vi "ImagerForFlowbit5.vi"() -> ()   [LabVIEW 2011]
uses:
  <vilib>/vision/Image Controls.llb/IMAQ Image.ctl
  <vilib>/Platform/TimedLoop/XDataNode/timing_clust.ctl
  <vilib>/Platform/TimedLoop/XDataNode/nitl_modes.ctl
  <vilib>/Platform/TimedLoop/XDataNode/wakeup.ctl
  <vilib>/Utility/config.llb/Read Key (I32).vi
  <vilib>/Analysis/1siggen.llb/Riffle Array (I32).vi
  <vilib>/Platform/TimedLoop/XDataNode/XDataNode.xnode
  <vilib>/Analysis/NI_AALBase.lvlib
  <vilib>/vision/NI_Vision_Development_Module.lvlib
  <vilib>/Platform/TimedLoop/XDataNode/XDNodeRunTimeDep.lvlib
  <vilib>/Utility/config.llb/NI_LVConfig.lvlib
panel:
  out "onLineMapOutput":T1[](array[typedef])
  out "Bounds.Right":i16
  out "停止循环":bool
  in  "Stimuli":i64=5
  in  "选项卡控件":enum32{"前面板", "参数设置", "OnLineMap"}(tab)
  out "log":string
  out "Stim_ID":i32(listbox)=1
  in  "开始/暂停":bool=TRUE
  in  "停止":bool
  out "重排的 Stim ID":i32[](array[numeric]) caption="重排的{X}"
  out "block":i32
  out "队列中元素数量":i32
  out "Image 2":T1(plugin-control)
  in  "热图":bool
  out "循环持续时间":i64
  out "Recording":bool
  out "grabLoop":i32
  out "writeing data":bool
  out "address":i16=888 caption="地址" format="%.0x"
  in  "SaveParameter":bool
  in  "Pra_binType":enum16{"Extract", "Resample"}(ring)
  in  "Pra_FramesPerStim":i64=16
  in  "Pra_Blk目录":path=path "D:/Expt/test"
  in  "Pra_文件名":string="G4_E02"
  in  "Pra_TimeForPrepare(ms)":u32=1000
  in  "Pra_stim ID":u8[](array[numeric])=[0, 2, 4, 6, 8]
  in  "Pra_blk总数":i32=500
  in  "Pra_stim protocol":T2(array[ring])=[enum."prep stim", enum."wait respirator", enum."show stim", enum."recording data", enum."Blank stim", enum."writing data", enum."ISI"]
  in  "Pra_blank stim":u8
  in  "Pra_wait（ms）":u32=10
  in  "Pra_ISI（ms）":u32=8000
  in  "Pra_FrameBin":i32=25
  in  "Pra_datatype":u16(ring)=13 items=["U8"=11, "I16"=12, "U32"=13, "SGL"=14]
  in  "FrameWidth":i64=704
  in  "FrameHeight":i64=576
  in  "LoadParameter":bool
  in  "Pra_bin":enum16{"1*1", "2*2"}(ring)
  in  "Pra_DR/R parameter":T3={"frame_zero_0"=0, "frame_zero_1"=1, "frame_0"=3, "frame_1"=15}
  in  "Pra_OnlineMap":cluster{"数组 1":i32[], "数组 2":i32[]}[](array[cluster])=[{"数组 1"=[2], "数组 2"=[6]}, {"数组 1"=[4], "数组 2"=[8]}, {"数组 1"=[2, 6], "数组 2"=[4, 8]}, {"数组 1"=[2, 4, 6, 8], "数组 2"=[0]}, {"数组 1"=[2, 4], "数组 2"=[6, 8]}]
  in  "Pra_clip ratio":dbl=2.0 min=0.0001 step=0.1
  # "-"
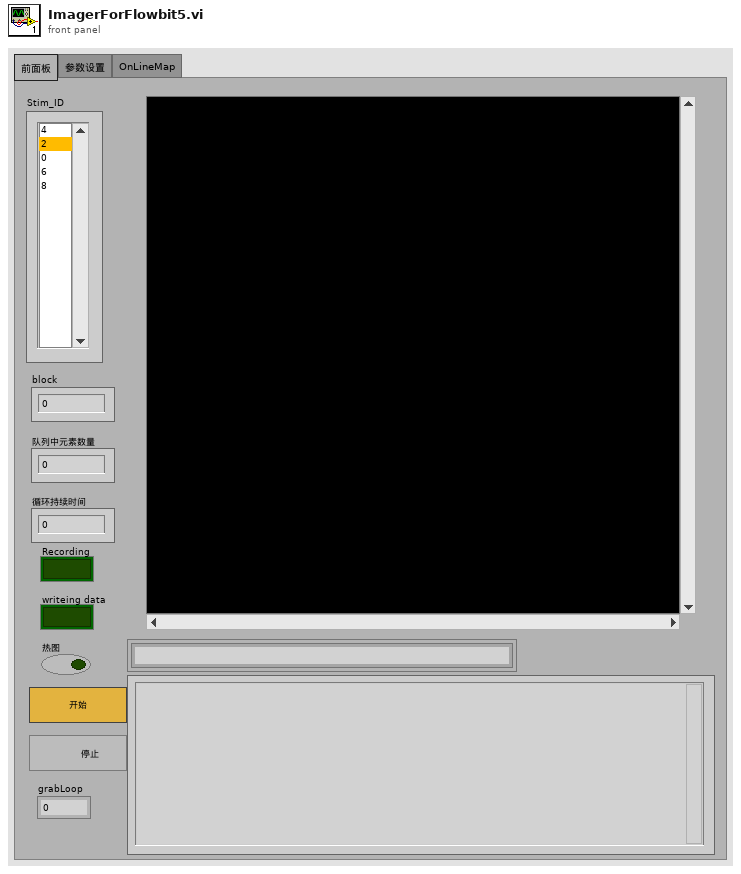
[diagram p1: front panel]
types:
  T1 = typedef "IMAQ Image.ctl" = refnum<image>
  T2 = enum16{"wait", "prep stim", "show stim", "wait respirator", "recording data", "Blank stim", "wait heart", "ISI", "DR/R", "wait calibrate", "openLightShutter", "closeLightShutter", "writing data"}[]
  T3 = cluster{"frame_zero_0":i32, "frame_zero_1":i32, "frame_0":i32, "frame_1":i32}
  T4 = typedef "Image Type" = u32
  T5 = enum16{"Disable External Trigger", "Enable External Trigger"}
  T6 = enum32{"Auto Detect", "RoadRunner", "Raven", "R64"}
  T7 = typedef "LVAllMonitorsDisplayTypeDef.ctl" = cluster{"Bounds":cluster{"Left":i16, "Top":i16, "Right":i16, "Bottom":i16}, "Depth":i16}[]
  T8 = cluster{"Bounds":cluster{"Left":i16, "Top":i16, "Right":i16, "Bottom":i16}, "Depth":i16}
  T9 = typedef "NI_LVConfig.lvlib/Config Data RefNum.ctl" = refnum<k1>
  T10 = enum16{"big-endian, network order", "native, host order", "little-endian"}
  T11 = enum8{"Enabled", "Disabled", "Disabled and Grayed Out"}
  T12 = enum16{"open", "replace", "create", "open or create", "replace or create", "replace or create with confirmation"}
  T13 = cluster{"Browser Size":cluster{"X":i32, "Y":i32}, "Images per Line":i32, "Background Color":u32, "Frame Size":i32, "Frame Style":enum16{"Raised", "Bevelled", "Outline", "Hidden", "Step", "Raised Outline"}}
  T14 = cluster{"Desired Font (Application)":enum16{"User-specified Font", "Application Font", "System Font", "Dialog Font"}, "[User-specified Font]":cluster{"Font Name":string, "Size":i16, "Strikeout?":bool, "Italic?":bool, "Underline?":bool, "Outline?":bool, "Shadow?":bool, "Bold?":bool, "Rotation Angle":dbl}, "Horizontal Alignment":i16, "Vertical Alignment":i16}
  T15 = typedef "XDNodeRunTimeDep.lvlib/timing_clust.ctl" = cluster{"Expected End [f-1]":u64, "Actual End [f-1]":u64, "Finished Late? [f-1]":bool, "Expected End [i-1]":u64, "Actual End [i-1]":u64, "Finished Late? [i-1]":bool, "Expected Start [i]":u64, "Actual Start [i]":u64, "Expected Start [f]":u64, "Actual Start [f]":u64, "Source Name":string, "Structure Name":string, "Period":i64, "Deadline":i64, "Offset":i64, "Start":i64, "Priority":i32, "Timeout":i32, "Mode":T16, "Wakeup Reason":T17, "Error":errorcluster, "Source Type":string, "Secondary Source Type":string, "Global End Time":u64, "Global Start Time":u64, "Frame Duration":u64, "Iteration Duration":u64, "Assigned CPU":i32, "I/O Scan Engine Mode":u32}
  T16 = typedef "XDNodeRunTimeDep.lvlib/nitl_modes.ctl" = enum32{"No Change", "Process missed periods, maintain original phase", "Discard missed periods, maintain original phase", "Process missed periods, ignore original phase", "Discard missed periods, ignore original phase"}
  T17 = typedef "XDNodeRunTimeDep.lvlib/wakeup.ctl" = enum32{"Normal", "Aborted", "Asynchronous wakeup", "Timing source error", "Timed loop error", "Timeout"}
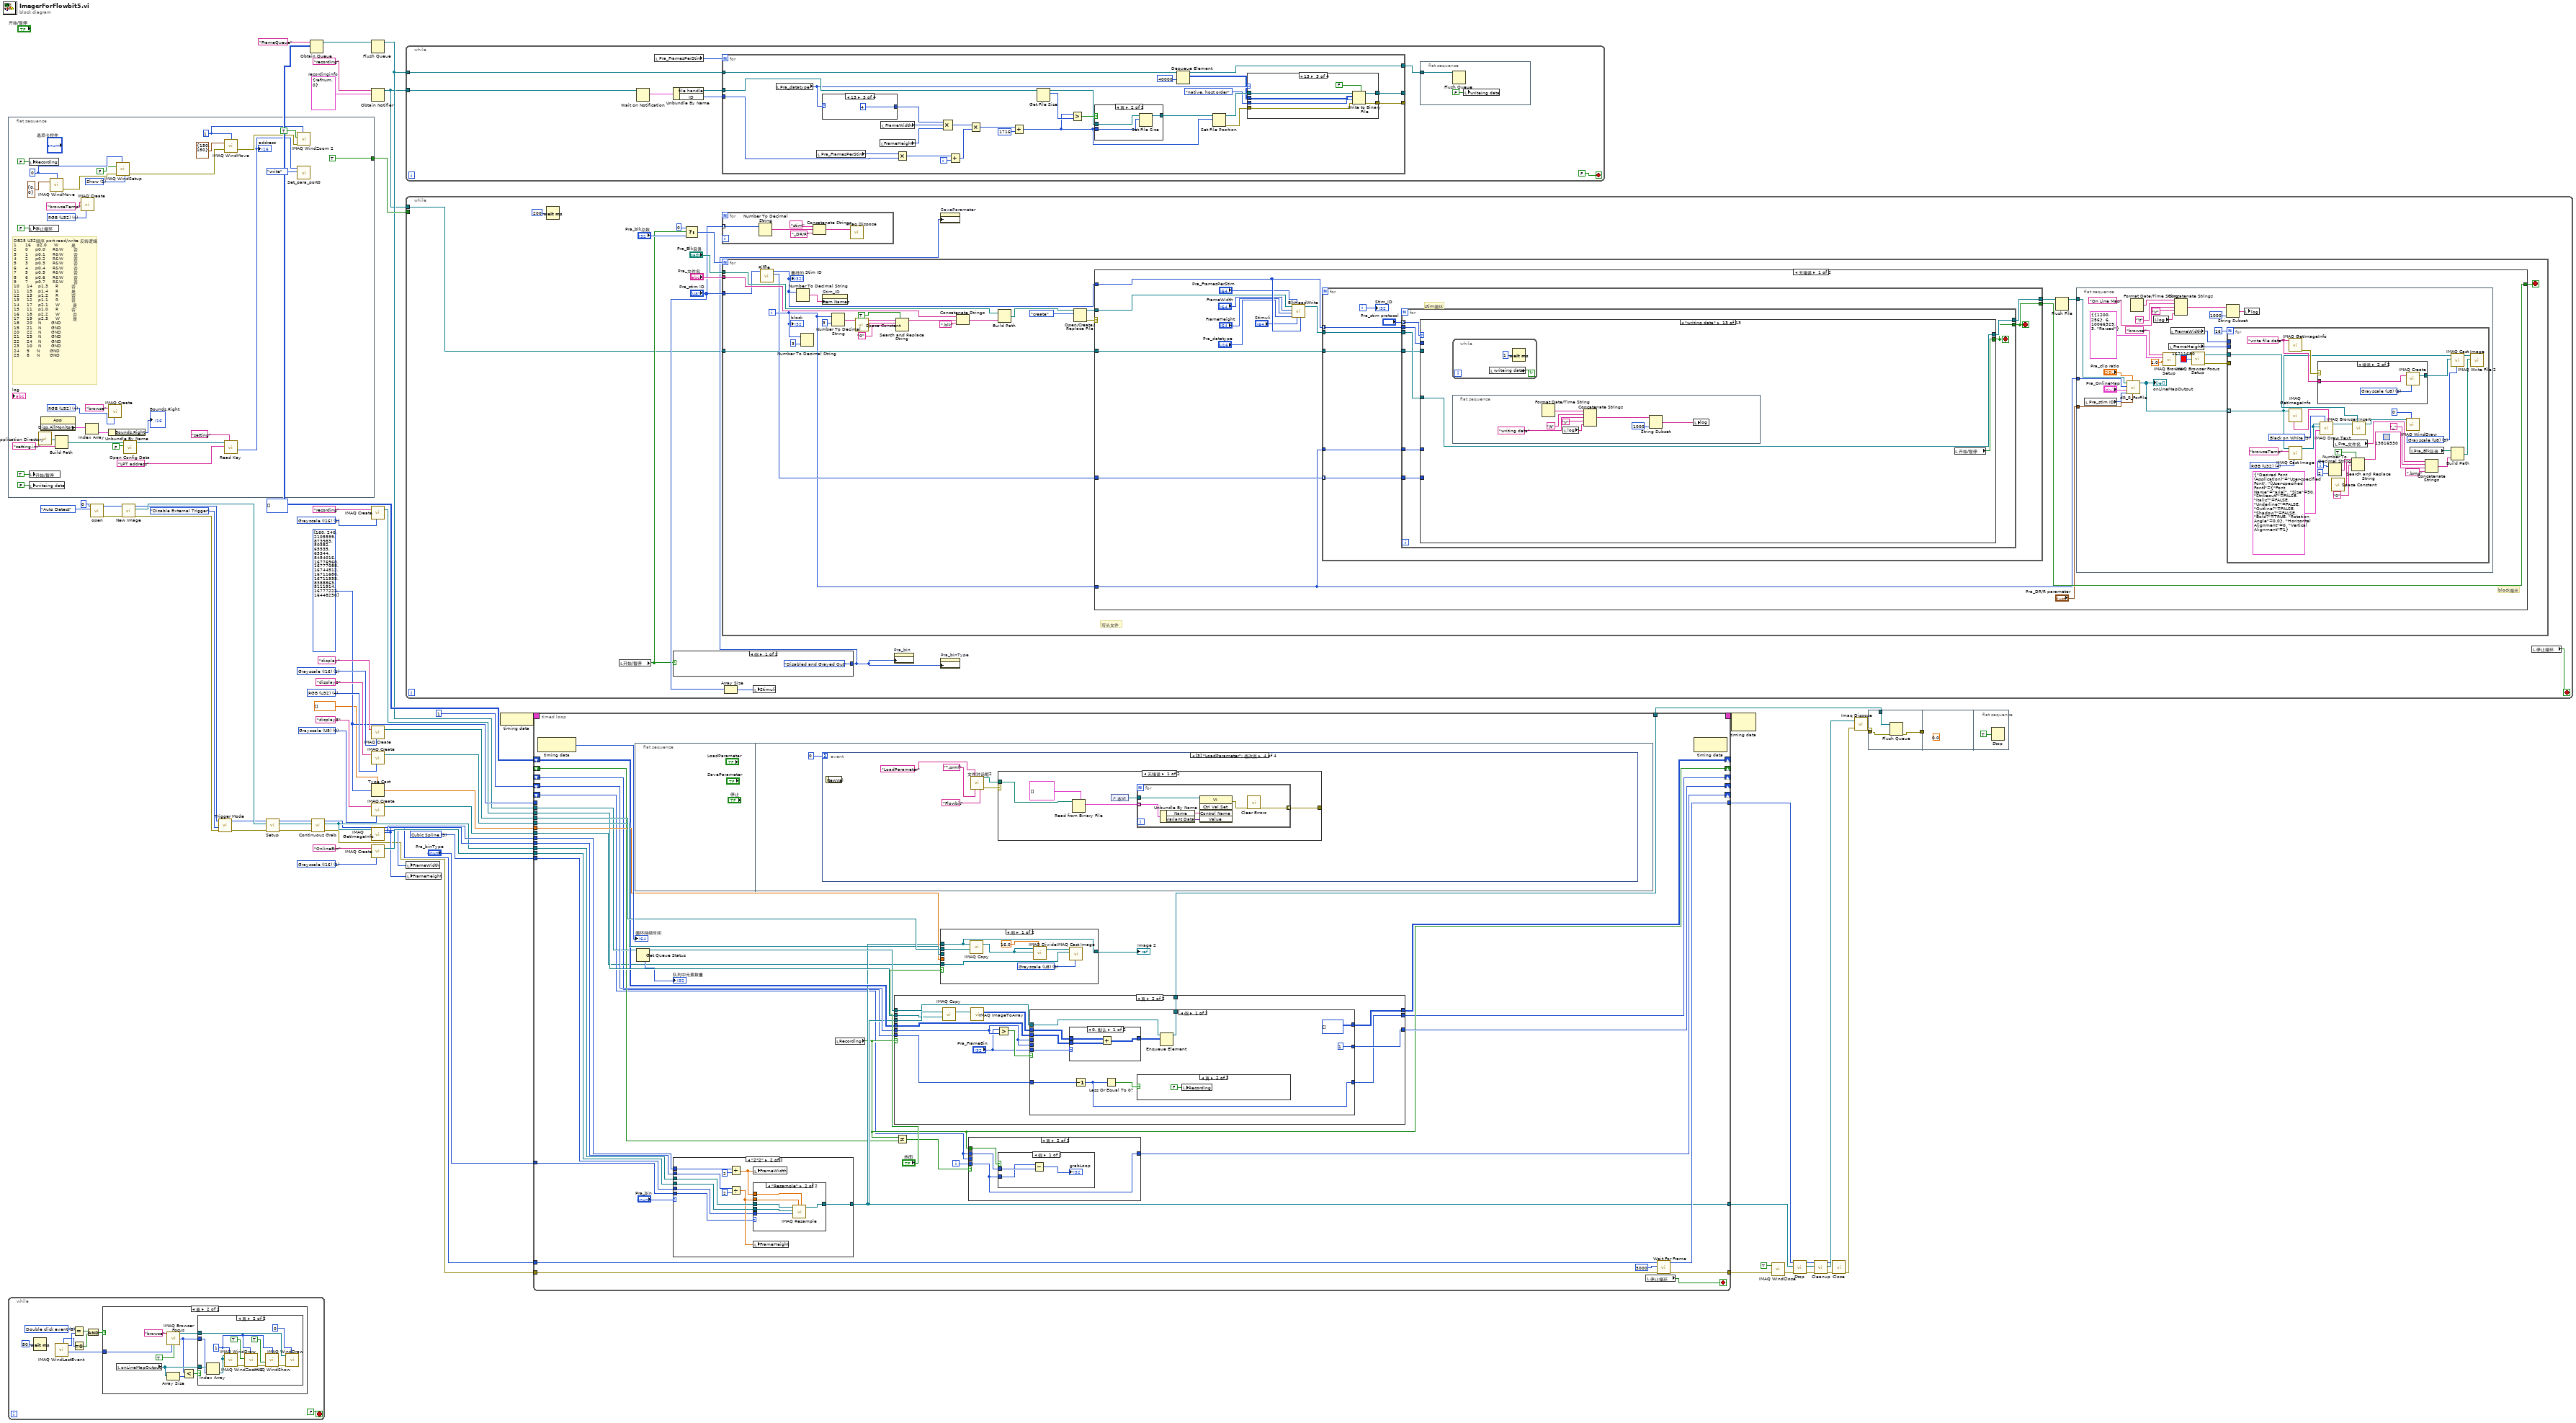
[diagram p0: block diagram]
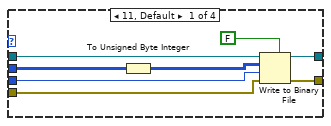
[diagram p4: hidden frame]
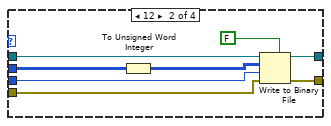
[diagram p5: hidden frame]
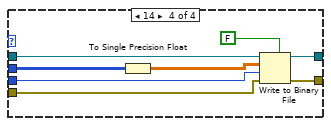
[diagram p6: hidden frame]
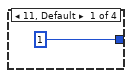
[diagram p8: hidden frame]
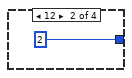
[diagram p9: hidden frame]
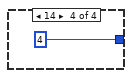
[diagram p10: hidden frame]
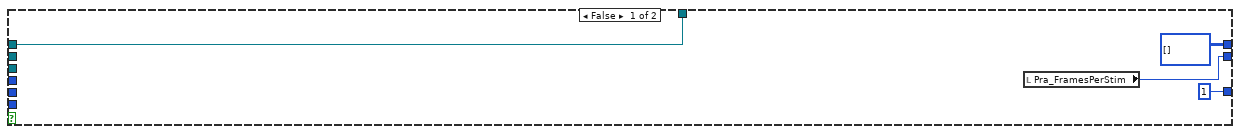
[diagram p11: hidden frame]
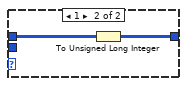
[diagram p13: hidden frame]
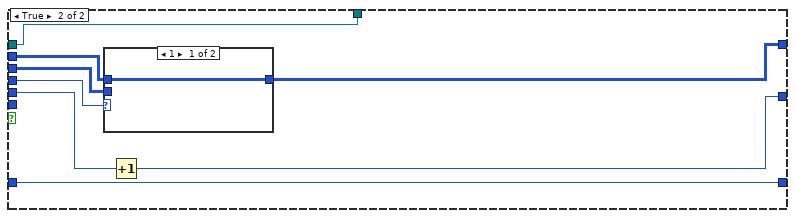
[diagram p14: hidden frame]
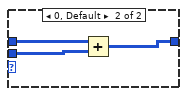
[diagram p15: hidden frame]
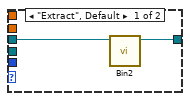
[diagram p19: hidden frame]
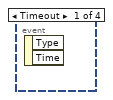
[diagram p20: hidden frame]
diagram:
  w10 = cluster{"file handle":refnum<file>, "ID":i32} {"file handle"=refnum, "ID"=0}  # recordinginfo
  w15 = T4 0 items=["Grayscale (U8)", "Grayscale (I16)", "Grayscale (SGL)", "Complex (CSG)", "RGB (U32)", "HSL (U32)", "RGB (U64)", "Grayscale (U16)"] ("Image Type")
  w20 = u32 3 items=["Zero Order", "Bi-Linear", "Quadratic", "Cubic Spline"] ("Interpolation Type")
  w22 = T4 1 items=["Grayscale (U8)", "Grayscale (I16)", "Grayscale (SGL)", "Complex (CSG)", "RGB (U32)", "HSL (U32)", "RGB (U64)", "Grayscale (U16)"] ("Image Type")
  w24 = u32[][] []
  w33 = T4 4 items=["Grayscale (U8)", "Grayscale (I16)", "Grayscale (SGL)", "Complex (CSG)", "RGB (U32)", "HSL (U32)", "RGB (U64)", "Grayscale (U16)"] ("Image Type")
  w31 = u32[] [160, 240, 2105599, 873983, 50382, 65535, 65344, 8454016, 16776960, 16777088, 16744512, 16711680, 16711935, 8388863, 5111914, 16777222, 16448250] ("数组")
  w37 = T4 1 items=["Grayscale (U8)", "Grayscale (I16)", "Grayscale (SGL)", "Complex (CSG)", "RGB (U32)", "HSL (U32)", "RGB (U64)", "Grayscale (U16)"] ("Image Type")
  w38 = T4 1 items=["Grayscale (U8)", "Grayscale (I16)", "Grayscale (SGL)", "Complex (CSG)", "RGB (U32)", "HSL (U32)", "RGB (U64)", "Grayscale (U16)"] ("Image Type")
  n1 = flat-sequence {
    tunnel: [TRUE ("Zoom to Fit Mode")] -> w26
    frame #0 {
      w70 = 1 items=["Hide", "Show", "No change"] ("Scrollbars (No change)")
      w67 = 1 ("Window Number (0...15)")
      w71 = 0 ("Window Number (0...15)")
      w76 = T4 4 items=["Grayscale (U8)", "Grayscale (I16)", "Grayscale (SGL)", "Complex (CSG)", "RGB (U32)", "HSL (U32)", "RGB (U64)", "Grayscale (U16)"] ("Image Type")
      w77 = T4 4 items=["Grayscale (U8)", "Grayscale (I16)", "Grayscale (SGL)", "Complex (CSG)", "RGB (U32)", "HSL (U32)", "RGB (U64)", "Grayscale (U16)"] ("Image Type")
      # "DB25\tU32顺序\tport\tread/write\t反转逻辑\n1\t     16\t   p2.0    \tW\t        是\n2\t     0    \tp0.0\t   \tR&W\t      否\n3\t     1\t\t   p0.1\t   \tR&W      \t否\n4\t\t    2\t   \tp0.2   \t\tR&W      \t否\n5\t\t    3\t\t   p0.3   \t\tR&W\t      否\n6\t\t    4\t   \tp0.4   \t\tR&W      \t否\n7\t\t    5\t   \tp0.5   \t\tR&W      \t否\n8\t\t    6\t   \tp0.6\t   \tR&W      \t否\n9\t    \t7\t   \tp0.7\t   \tR&W\t      否\n10\t    14   \tp1.3   \t\tR        \t否\n11\t   \t15   \tp1.4   \t\tR        \t是\n12\t   \t13   \tp1.2\t   \tR        \t否\n13    \t12   \tp1.1\t   \tR        \t否\n14     17   \tp2.1\t   \tW        \t是\n15    \t11   \tp1.0   \t\tR\t        否\n16    \t18   \tp2.2   \t\tW        \t否\n17    \t19\t   p2.3   \t\tW\t        是\n18    \t20   \tN   \t  \tGND\t\n19    \t21   \tN   \t  \tGND\t\n20\t    22\t   N\t  \t  \tGND\t\n21\t    23\t   N  \t  \t\tGND\t\n22\t    24\t   N  \t  \t\tGND\t\n23    \t10   \tN  \t  \t\tGND\t\n24    \t9\t    N  \t  \t\tGND\t\n25\t    8    \tN  \t  \t\tGND"
      n2 = local write "Recording"(FALSE ("Recording")) -> ()
      n3 = local write "停止循环"(FALSE ("开始/暂停")) -> ()
      n4 = local write "开始/暂停"(TRUE ("开始/暂停")) -> ()
      n5 = local write "writeing data"(FALSE ("Recording")) -> ()
      n6 = call <vilib>:"Application Directory.vi"() -> ("Application Directory"=w89:path)
      n7 = property class="App"() -> ("Disp.AllMonitors"=w81:T7)  [unwired: 2 in, 2 out]
      n8 = call "IMAQ WindMove"("Window Number (0...15)"=w71, "Coordinates (screen)"=cluster{"X Position":i32, "Y Position":i32} {"X Position"=0, "Y Position"=0}) -> ("error out"=w72:errorcluster)  [unwired: 3 in, 1 out]
      n9 = Build Path(base path=w89, name or relative path="setting.ini" ("名称或相对路径")) -> (appended path=w87:path)
      n10 = call "IMAQ Create"("Image Name"="browseTemp", "Image Type"=w76) -> ()  [unwired: 3 in, 2 out]
      n11 = Index Array(array=w81) -> (element=w80:T8)  [unwired: 1 in]
      n12 = call "IMAQ Create"("Image Name"="browse", "Image Type"=w77) -> ()  [unwired: 3 in, 2 out]
      n13 = Unbundle By Name(w80) -> ("Bounds.Right"=→"Bounds.Right":i16)
      n14 = call "IMAQ WindSetup"("Scrollbars (No change)"=w70, "Window Number (0...15)"=w71, "error in (no error)"=w72, "Window can close? (Yes)"=FALSE) -> ("error out"=w69:errorcluster)  [unwired: 7 in]
      n15 = call <vilib>:"Open Config Data.vi"("create file if necessary (T)"=FALSE, "configuration file path"=w87) -> ("refnum"=w85:T9)  [unwired: 7 in, 2 out]
      n16 = call "IMAQ WindMove"("Window Number (0...15)"=w67, "Coordinates (screen)"=cluster{"X Position":i32, "Y Position":i32} {"X Position"=150, "Y Position"=150}, "error in (no error)"=w69) -> ("error out"=w68:errorcluster)  [unwired: 2 in, 1 out]
      n17 = call-poly <vilib>:"Read Key.vi"("section"="setting", "key"="LPT address", "refnum"=w85) -> ("value"=w82:i32)  [unwired: 5 in, 3 out]
      "address" <- w82
      n18 = call "IMAQ WindZoom 2"("Window Number (0...15)"=w67, "error in (no error)"=w68, "Zoom to Fit? (False)"=TRUE) -> ()  [unwired: 5 in, 4 out]
      n19 = call "Set_para_port0.vi"("R or W"=enum16{"read", "write"}."write", "address"=w82) -> ()  [unwired: 8 in, 2 out]
    }
  }
  n20 = while {
    stop <- FALSE stop-if-true
    w102 = 8 items=["No  event", "Click event", "Draw event", "Move event", "Size event", "Scroll event", "Activate event", "Close event", "Double click event"] ("Event")
    n21 = Wait (ms)(milliseconds to wait=u32 50 ("等待时间（毫秒）")) -> ()  [unwired: 1 out]
    n22 = call "IMAQ WindLastEvent"() -> ("Coordinates"=w96:i32[], "Event"=w101:i32, "Window Number (0...15)"=w100:i32)  [unwired: 6 in, 3 out]
    n23 = Equal?(x=w102, y=w101) -> (x = y?=w99:bool)
    n24 = Equal To 0?(x=w100) -> (x = 0?=w98:bool)
    n25 = And(x=w99, y=w98) -> (x .and. y?=w97:bool)
    n26 = case shown="真" w97 {
      tunnel: w96 -> [_ w112]
      frame False {
      }
      frame True {
        n27 = local read "onLineMapOutput"() -> (w108:T1[])
        n28 = call "IMAQ Browser Focus"("Image Browser In"="browse" ("Image Name"), "Pixel Position"=w112, "Get/Set (Set)"=TRUE) -> ("Image Browser Out"=w106:T1, "Index Out"=w107:i32)  [unwired: 5 in, 6 out]
        n29 = Array Size(array=w108) -> (size(s)=w110:i32)
        n30 = Less?(x=w107, y=w110) -> (x < y?=w109:bool)
        n31 = case shown="真" w109 {
          tunnel: w108 -> [_ w123]
          tunnel: w107 -> [_ w122]
          tunnel: w106 -> [_ w120]
          frame False {
          }
          frame True {
            w114 = 1 ("Window Number (0...15)")
            n32 = Index Array(array=w123, index=w122) -> (element=w121:T1)
            n33 = call "IMAQ WindDraw"("Window Number (0...15)"=w114, "Title"=w121, "Image"=w121) -> ("error out"=w117:errorcluster)  [unwired: 7 in, 1 out]
            n34 = call "IMAQ WindZoom 2"("Window Number (0...15)"=w114, "error in (no error)"=w117, "Zoom to Fit? (False)"=TRUE) -> ("error out"=w116:errorcluster)  [unwired: 5 in, 3 out]
            n35 = call "IMAQ WindShow"("error in (no error)"=w116, "Bring To Front? (N)"=TRUE, "Window Number (0...15)"=w114) -> ("error out"=w115:errorcluster)  [unwired: 3 in, 2 out]
            n36 = call "IMAQ WindDraw"("Window Number (0...15)"=0, "error in (no error)"=w115, "Image"=w120) -> ()  [unwired: 7 in, 2 out]
          }
        }
      }
    }
  }
  n37 = call <vilib>:"open.vi"("Board Type"=T6."Auto Detect", "Board Number"=u32 0) -> ("error out"=w52:errorcluster, "RefBrdOut"=w48:u32)  [unwired: 2 in, 5 out]
  n38 = call <vilib>:"New Image.vi"("RefBrdIn"=w48, "error in"=w52) -> ("RefBrdOut"=w47:u32, "Image"=w60:T1, "error out"=w53:errorcluster)  [unwired: 6 in]
  n39 = call <vilib>:"Trigger Mode.vi"("RefBrdIn"=w47, "Trigger Mode"=T5."Disable External Trigger", "error in (no error)"=w53) -> ("RefBrdOut"=w46:u32, "error out"=w54:errorcluster)  [unwired: 6 in]
  n40 = call <vilib>:"Setup.vi"("error in"=w54, "Image In"=w60, "RefBrdIn"=w46) -> ("error out"=w49:errorcluster, "Image"=w50:T1, "RefBrdOut"=w45:u32)  [unwired: 6 in]
  n41 = Obtain Queue(name (unnamed)="FrameQueue" ("名称（未命名）"), element data type=w24) -> (queue out=w27:refnum<queue>)  [unwired: 3 in, 2 out]
  n42 = call <vilib>:"Continuous Grab.vi"("error in (no error)"=w49, "Image In"=w50, "RefBrdIn"=w45) -> ("error out"=w4:errorcluster, "Image"=w16:T1, "RefBrdOut"=w5:u32)  [unwired: 6 in]
  n43 = Flush Queue(queue=w27) -> (queue out=w12:refnum<queue>)  [unwired: 1 in, 2 out]
  n44 = Obtain Notifier(name (unnamed)="recording" ("名称（未命名）"), notification data type=w10) -> (notifier out=w9:refnum<notifier>)  [unwired: 2 in, 2 out]
  n45 = call "IMAQ Create"("Image Name"="recording", "Image Type"=w38) -> ("New Image"=w40:T1)  [unwired: 3 in, 1 out]
  n46 = call "IMAQ Create"("Image Name"="display", "Image Type"=w37) -> ("New Image"=w35:T1)  [unwired: 3 in, 1 out]
  n47 = call "IMAQ Create"("Image Name"="display2", "Image Type"=w33) -> ("New Image"=w32:T1)  [unwired: 3 in, 1 out]
  n48 = Type Cast(type=sgl[] [] ("单精度浮点"), x=w31) -> (*(type *) &x=w29:sgl[])
  n49 = call "IMAQ Create"("Image Name"="display3", "Image Type"=w15) -> ("New Image"=w13:T1)  [unwired: 3 in, 1 out]
  n50 = call "IMAQ GetImageInfo"("Image"=w16) -> ("Y Resolution"=w18:i32, "X Resolution"=w19:i32)  [unwired: 3 in, 6 out]
  n51 = call "IMAQ Create"("Image Name"="OnlineBin", "Image Type"=w22) -> ("New Image"=w21:T1)  [unwired: 3 in, 1 out]
  n52 = while {
    tunnel: w12 -> [w130]
    tunnel: w9 -> [w128]
    stop <- FALSE stop-if-true
    n53 = Wait on Notification(notifier=w128) -> (notification=w127:cluster{"file handle":refnum<file>, "ID":i32})  [unwired: 3 in, 3 out]
    n54 = local read "Pra_FramesPerStim"() -> (w129:i64)
    n55 = Unbundle By Name(w127) -> ("file handle"=w126:refnum<file>, "ID"=w125:i32)
    n56 = for {
      N: w129 -> [_]
      tunnel: w126 -> [w160]
      tunnel: w125 -> [w144]
      tunnel: [w152] -> _
      tunnel: [w151] -> w124
      tunnel: w130 -> [w136]
      tunnel: [w134] -> _
      i -> [w142]
      n57 = local read "Pra_datatype"() -> (w156:u16)
      n58 = local read "Pra_FramesPerStim"() -> (w145:i64)
      n59 = case shown="13" w156 {
        tunnel: [i64 1 i64 2 i64 4 i64 4] -> w148
        frame 11, Default {
        }
        frame 12 {
        }
        frame 13 {
        }
        frame 14 {
        }
      }
      n60 = local read "FrameHeight"() -> (w146:i64)
      n61 = local read "FrameWidth"() -> (w147:i64)
      n62 = Multiply(x=w145, y=w144) -> (x*y=w143:i64)
      n63 = Compound Arithmetic op=MULTIPLY(w148, w147, w146) -> (w140:i64)
      n64 = Add(x=w143, y=w142) -> (x+y=w141:i64)
      n65 = Multiply(x=w140, y=w141) -> (x*y=w139:i64)
      n66 = Add(x=w139, y=i64 1716 ("x")) -> (x+y=w137:i64)
      n67 = Get File Size(file=w160) -> (refnum out=w153:refnum<file>, size (in bytes)=w149:i64)  [unwired: 1 in, 1 out]
      n68 = Greater?(x=w137, y=w149) -> (0:w154:bool)
      n69 = case shown="真" w154 {
        tunnel: w137 -> [_ w195]
        tunnel: w153 -> [w192 w194]
        tunnel: [w192 w193] -> w155
        frame False {
        }
        frame True {
          n70 = Set File Size(6:w195, 7:w194) -> (3:w193:refnum<file>)  [unwired: 1 in, 1 out]
        }
      }
      n71 = Dequeue Element(queue=w136, timeout in ms (-1)=40000 ("超时毫秒(-1)")) -> (queue out=w151:refnum<queue>, element=w135:u32[][])  [unwired: 1 in, 2 out]
      n72 = Set File Position(offset (in bytes) (0)=w137, refnum=w155) -> (refnum out=w159:refnum<file>, error out=w157:errorcluster)  [unwired: 2 in]
      n73 = case shown="13" w156 {
        tunnel: w135 -> [w163 w172 w178 w185]
        tunnel: w159 -> [w167 w173 w181 w187]
        tunnel: T10."native, host order" ("字节顺序(0:big-endian, network order)") -> [w166 w174 w179 w188]
        tunnel: w157 -> [w165 w169 w180 w189]
        tunnel: [w164 w175 w182 w190] -> w152
        tunnel: [w161 w170 w177 w184] -> w134
        frame 11, Default {
          n74 = To Unsigned Byte Integer(number=w163) -> (unsigned 8bit integer=w162:u8[][])
          n75 = Write to Binary File(file (use dialog)=w167, data=w162, error in=w165, 5:FALSE ("预置数组或字符串大小？(T)"), 9:w166) -> (refnum out=w164:refnum<file>, error out=w161:errorcluster)  [unwired: 1 in, 1 out]
        }
        frame 12 {
          n76 = To Unsigned Word Integer(number=w172) -> (unsigned 16bit integer=w171:u16[][])
          n77 = Write to Binary File(file (use dialog)=w173, data=w171, error in=w169, 5:FALSE ("预置数组或字符串大小？(T)"), 9:w174) -> (refnum out=w175:refnum<file>, error out=w170:errorcluster)  [unwired: 1 in, 1 out]
        }
        frame 13 {
          n78 = Write to Binary File(file (use dialog)=w181, data=w178, error in=w180, 5:FALSE ("预置数组或字符串大小？(T)"), 9:w179) -> (refnum out=w182:refnum<file>, error out=w177:errorcluster)  [unwired: 1 in, 1 out]
        }
        frame 14 {
          n79 = To Single Precision Float(number=w185) -> (single precision float=w186:sgl[][])
          n80 = Write to Binary File(file (use dialog)=w187, data=w186, error in=w189, 5:FALSE ("预置数组或字符串大小？(T)"), 9:w188) -> (refnum out=w190:refnum<file>, error out=w184:errorcluster)  [unwired: 1 in, 1 out]
        }
      }
    }
    n81 = flat-sequence {
      tunnel: w124 -> [w133]
      frame #0 {
        n82 = Flush Queue(queue=w133) -> ()  [unwired: 1 in, 3 out]
        n83 = local write "writeing data"(FALSE ("writeing data")) -> ()
      }
    }
  }
  n84 = while {
    tunnel: w26 -> [_]
    tunnel: w9 -> [w200]
    stop <- w210 stop-if-true
    n85 = Wait (ms)(milliseconds to wait=u32 200 ("等待时间（毫秒）")) -> ()  [unwired: 1 out]
    n86 = local read "开始/暂停"() -> (w202:bool)
    n87 = case shown="假" w202 {
      tunnel: [T11."Disabled and Grayed Out" ("禁用") T11."Enabled" ("禁用")] -> w201
      frame False {
      }
      frame True {
      }
    }
    n88 = Select(t=0, s=w202, f="Pra_blk总数") -> (s? t:f=w207:i32)
    n89 = for {
      tunnel: "Pra_stim ID" -> [w215] mode=indexing
      n90 = Number To Decimal String(number=w215) -> (decimal integer string=w216:string)  [unwired: 1 in]
      n91 = Concatenate Strings("stim" ("字符串"), w216, "_DR/R" ("字符串")) -> (w214:string)
      n92 = call "Imaq Dispose"("Image"=w214) -> ()  [unwired: 5 in, 1 out]
    }
    n93 = for {
      N: w207 -> [_]
      tunnel: "Pra_stim ID" -> [w236]
      tunnel: "Pra_文件名" -> [w240]
      tunnel: "Pra_Blk目录" -> [w239]
      tunnel: w200 -> [w232]
      i -> [w234]
      stop <- w237 stop-if-true
      # "写头文件"
      n94 = call-poly <vilib>:"Riffle.vi"("X"=w236) -> ("Riffled Index"=w235:i32[], "Riffled {X}"=w238:i32[])  [unwired: 8 in, 1 out]
      "重排的 Stim ID" <- w238
      n95 = Number To Decimal String(number=w238) -> (decimal integer string=w222:string[])  [unwired: 1 in]
      n96 = Number To Decimal String(number=w234, width (-)=i16 3 ("宽度(-)")) -> ()  [unwired: 1 out]
      n97 = property on="Stim_ID" class="LstBox (严格)"("Item Names"=w222) -> ()  [unwired: 2 in, 2 out]
      n98 = Number To Decimal String(number=w234, width (-)=i16 3 ("宽度(-)")) -> (decimal integer string=w227:string)
      n99 = call <vilib>:"Space Constant.vi"() -> ("String"=w228:string)
      n100 = Search and Replace String(replace all?=TRUE ("替换全部？(F)"), input string=w227, search string=w228, replace string="0" ("替换字符串(\"\")")) -> (result string=w225:string)  [unwired: 4 in, 3 out]
      n101 = Concatenate Strings(w240, w225, ".blk" ("字符串")) -> (w223:string)
      n102 = Build Path(base path=w239, name or relative path=w223) -> (appended path=w233:path)
      n103 = Open/Create/Replace File(file path (use dialog)=w233, operation (0:open)=T12."create" ("操作(0:open)")) -> (refnum out=w220:refnum<file>, error out=w219:errorcluster)  [unwired: 4 in, 1 out]
      n104 = case shown="无错误" w219 {
        tunnel: w238 -> [w254 _]
        tunnel: [w253 TRUE ("开始/暂停")] -> w237
        tunnel: w235 -> [w252 _]
        tunnel: w234 -> [w250 _]
        tunnel: w232 -> [w247 _]
        tunnel: w220 -> [w242 _]
        frame No Error {
          # "block循环"
          n105 = call "BlkHeadWrite.vi"("SequenceOfID"=w254, "Stimuli"="Stimuli", "FramesPerStim"="Pra_FramesPerStim", "datatype"="Pra_datatype", "FrameHeight"="FrameHeight", "FrameWidth"="FrameWidth", "引用句柄输入"=w242) -> ("引用句柄输出"=w255:refnum<file>)  [unwired: 4 in]
          n106 = for {
            tunnel: w255 -> [w322]
            tunnel: [w320] -> w249
            tunnel: w252 -> [w321] mode=indexing
            tunnel: w254 -> [w319] mode=indexing
            tunnel: [w318] -> w253
            tunnel: w250 -> [w315]
            tunnel: w247 -> [w314]
            i -> [w317]
            stop <- w318 stop-if-true
            # "stim循环"
            n107 = for {
              tunnel: w321 -> [w329]
              tunnel: w319 -> [w327]
              tunnel: [w325] -> w318
              tunnel: "Pra_stim protocol" -> [w326] mode=indexing
              tunnel: w322 -> [w330]
              tunnel: [w328] -> w320
              tunnel: w315 -> [w324]
              tunnel: w314 -> [w323]
              stop <- w325 stop-if-true
              n108 = case shown="\"writing data\"" w326 {
                tunnel: w330 -> [w333 w353 w368 w382 w399 w412 w426 w441 w463 w473 w475 w488 w501]
                tunnel: w329 -> [_ _ _ w384 _ _ _ w439 _ _ _ _ _]
                tunnel: [w333 w353 w368 w382 w399 w412 w426 w441 w463 w473 w475 w488 w501] -> w328
                tunnel: w327 -> [w331 _ _ _ _ _ _ _ _ _ _ _ _]
                tunnel: [w334 w354 w369 w381 w400 w413 w427 w440 w464 w474 w476 w489 w502] -> w325
                tunnel: w324 -> [_ _ _ _ _ _ _ w438 _ _ _ _ _]
                tunnel: w323 -> [_ _ _ w385 _ _ _ _ _ _ _ _ _]
                frame "prep stim" {
                  n109 = Number To Boolean Array(number=w331) -> (Boolean array=w335:bool[])
                  n110 = flat-sequence {
                    tunnel: w335 -> [w346]
                    tunnel: [w346] -> w332
                    tunnel: w331 -> [w345]
                    tunnel: w332 -> [w351]
                    frame #0 {
                      n111 = Number To Decimal String(number=w345) -> (decimal integer string=w342:string)  [unwired: 1 in]
                      n112 = Format Date/Time String() -> (date/time string=w344:string)  [unwired: 3 in]
                      n113 = local read "log"() -> (w338:string)
                      n114 = Concatenate Strings(w344, "\t", "prep stim ID=" ("字符串"), w342, "\r", w338) -> (w340:string)
                      n115 = String Subset(string=w340, length (rest)=1000 ("y")) -> (substring=w339:string)  [unwired: 1 in]
                      n116 = local write "log"(w339) -> ()
                    }
                    frame #1 {
                      n117 = local read "address"() -> (w348:i16)
                      n118 = local read "address"() -> (w347:i16)
                      n119 = call "Write_para_port0.vi"("port0（8元素）"=w351, "address"=w347) -> ()  [unwired: 9 in, 1 out]
                      n120 = call "Write_para_port2_singalChange.vi"("索引"=0, "布尔"=TRUE, "address"=w348) -> ()  [unwired: 8 in, 1 out]
                    }
                    frame #2 {
                      n121 = Wait (ms)(milliseconds to wait="Pra_TimeForPrepare(ms)") -> ()  [unwired: 1 out]
                    }
                  }
                  n122 = local read "开始/暂停"() -> (w334:bool)
                }
                frame "wait respirator" {
                  n123 = while {
                    stop <- w365 stop-if-true
                    # "this step will return true if pallel port doesn't connect any signal.That means this loop only run once."
                    n124 = Wait (ms)(milliseconds to wait=u32 5 ("等待时间（毫秒）")) -> ()  [unwired: 1 out]
                    n125 = local read "address"() -> (w363:i16)
                    n126 = call "read_para_port1.vi"("address"=w363) -> ("port1（5元素）"=w367:bool[])  [unwired: 9 in, 1 out]
                    n127 = Index Array(array=w367, index=3 ("索引")) -> (element=w365:bool)
                  }
                  n128 = flat-sequence {
                    frame #0 {
                      n129 = Format Date/Time String() -> (date/time string=w362:string)  [unwired: 3 in]
                      n130 = local read "log"() -> (w357:string)
                      n131 = Concatenate Strings(w362, "\t", "wait respiratory" ("字符串"), "\r", w357) -> (w359:string)
                      n132 = String Subset(string=w359, length (rest)=1000 ("y")) -> (substring=w358:string)  [unwired: 1 in]
                      n133 = local write "log"(w358) -> ()
                    }
                  }
                  n134 = local read "开始/暂停"() -> (w354:bool)
                }
                frame "show stim" {
                  n135 = flat-sequence {
                    frame #0 {
                      n136 = local read "address"() -> (w378:i16)
                      n137 = call "Write_para_port2_singalChange.vi"("索引"=0, "布尔"=FALSE, "address"=w378) -> ()  [unwired: 8 in, 1 out]
                    }
                  }
                  n138 = flat-sequence {
                    frame #0 {
                      n139 = Format Date/Time String() -> (date/time string=w377:string)  [unwired: 3 in]
                      n140 = local read "log"() -> (w372:string)
                      n141 = Concatenate Strings(w377, "\t", "show stim" ("字符串"), "\r", w372) -> (w374:string)
                      n142 = String Subset(string=w374, length (rest)=1000 ("y")) -> (substring=w373:string)  [unwired: 1 in]
                      n143 = local write "log"(w373) -> ()
                    }
                  }
                  n144 = local read "开始/暂停"() -> (w369:bool)
                }
                frame "recording data" {
                  n145 = flat-sequence {
                    frame #0 {
                      n146 = Format Date/Time String() -> (date/time string=w397:string)  [unwired: 3 in]
                      n147 = local read "log"() -> (w392:string)
                      n148 = Concatenate Strings(w397, "\t", "recording data" ("字符串"), "\r", w392) -> (w394:string)
                      n149 = String Subset(string=w394, length (rest)=1000 ("y")) -> (substring=w393:string)  [unwired: 1 in]
                      n150 = local write "log"(w393) -> ()
                    }
                  }
                  n151 = flat-sequence {
                    frame #0 {
                      "Recording" <- TRUE ("Recording")
                      "writeing data" <- TRUE ("Recording")
                    }
                    frame #1 {
                      n152 = while {
                        stop <- w389 continue-if-true
                        n153 = local read "Recording"() -> (w389:bool)
                        n154 = Wait (ms)(milliseconds to wait=u32 1 ("等待时间（毫秒）")) -> ()  [unwired: 1 out]
                      }
                    }
                  }
                  n155 = Bundle("引用句柄输出"=w382, w384) -> (w383:cluster{"引用句柄输出":refnum<file>, i32})  [unwired: 1 in]
                  n156 = Send Notification(notification=w383, notifier=w385) -> ()  [unwired: 1 in, 2 out]
                  n157 = local read "开始/暂停"() -> (w381:bool)
                }
                frame "Blank stim" {
                  n158 = flat-sequence {
                    frame #0 {
                      n159 = Format Date/Time String() -> (date/time string=w410:string)  [unwired: 3 in]
                      n160 = local read "log"() -> (w405:string)
                      n161 = Concatenate Strings(w410, "\t", "show blank stim" ("字符串"), "\r", w405) -> (w407:string)
                      n162 = String Subset(string=w407, length (rest)=1000 ("y")) -> (substring=w406:string)  [unwired: 1 in]
                      n163 = local write "log"(w406) -> ()
                    }
                  }
                  n164 = local read "address"() -> (w398:i16)
                  n165 = Number To Boolean Array(number="Pra_blank stim") -> (Boolean array=w401:bool[])
                  n166 = call "Write_para_port0.vi"("port0（8元素）"=w401, "address"=w398) -> ()  [unwired: 9 in, 1 out]
                  n167 = local read "开始/暂停"() -> (w400:bool)
                }
                frame "ISI" {
                  n168 = flat-sequence {
                    tunnel: "Pra_ISI（ms）" -> [w417]
                    tunnel: "Pra_ISI（ms）" -> [w424]
                    frame #0 {
                      n169 = Number To Decimal String(number=w417) -> (decimal integer string=w421:string)  [unwired: 1 in]
                      n170 = Format Date/Time String() -> (date/time string=w423:string)  [unwired: 3 in]
                      n171 = local read "log"() -> (w416:string)
                      n172 = Concatenate Strings(w423, "\t", "ISI(ms)=" ("字符串"), w421, "\r", w416) -> (w419:string)
                      n173 = String Subset(string=w419, length (rest)=1000 ("y")) -> (substring=w418:string)  [unwired: 1 in]
                      n174 = local write "log"(w418) -> ()
                    }
                    frame #1 {
                      n175 = Wait (ms)(milliseconds to wait=w424) -> ()  [unwired: 1 out]
                    }
                  }
                  n176 = local read "开始/暂停"() -> (w413:bool)
                }
                frame "wait", Default {
                  n177 = Wait (ms)(milliseconds to wait="Pra_wait（ms）") -> ()  [unwired: 1 out]
                  n178 = flat-sequence {
                    tunnel: "Pra_wait（ms）" -> [w431]
                    frame #0 {
                      n179 = Number To Decimal String(number=w431) -> (decimal integer string=w435:string)  [unwired: 1 in]
                      n180 = Format Date/Time String() -> (date/time string=w437:string)  [unwired: 3 in]
                      n181 = local read "log"() -> (w430:string)
                      n182 = Concatenate Strings(w437, "\t", "wait(ms)=" ("字符串"), w435, "\r", w430) -> (w433:string)
                      n183 = String Subset(string=w433, length (rest)=1000 ("y")) -> (substring=w432:string)  [unwired: 1 in]
                      n184 = local write "log"(w432) -> ()
                    }
                  }
                  n185 = local read "开始/暂停"() -> (w427:bool)
                }
                frame "DR/R" {
                  n186 = disable-structure shown="禁用" {
                    frame Disabled {
                      n187 = flat-sequence {
                        frame #0 {
                          n188 = Format Date/Time String() -> (date/time string=w449:string)  [unwired: 3 in]
                          n189 = local read "log"() -> (w444:string)
                          n190 = Concatenate Strings(w449, "\t", "DR/R" ("字符串"), "\r", w444) -> (w446:string)
                          n191 = String Subset(string=w446, length (rest)=1000 ("y")) -> (substring=w445:string)  [unwired: 1 in]
                          n192 = local write "log"(w445) -> ()
                        }
                      }
                    }
                    frame Enabled {
                    }
                  }
                  n193 = disable-structure shown="禁用" {
                    disable-tunnel: w439 -> [w454 _]
                    disable-tunnel: w438 -> [w453 _]
                    frame Disabled {
                      n194 = local read item#-1() -> (w450)
                      n195 = Index Array(array=w450, index=w454) -> (element=w451)
                      n196 = call "dR.vi"() -> ("Image Dst Out"=w452:T1)  [unwired: 11 in]
                      n197 = case shown="0" w453 {
                        selector: w453 -> [_ w459]
                        tunnel: w452 -> [w456 w460]
                        tunnel: w451 -> [w455 w462]
                        frame 0 {
                          n198 = call "IMAQ Copy"("Image Dst"=w455, "Image Src"=w456) -> ()  [unwired: 4 in, 2 out]
                        }
                        frame 1, Default {
                          n199 = Increment(x=w459) -> (x+1=w458:i32)
                          n200 = call "IMAQ Multiply"("Image Src A"=w462, "Constant"=w459, "Image Dst"=w462) -> ("Image Dst Out"=w461:T1)  [unwired: 4 in, 1 out]
                          n201 = call "IMAQ Add"("Image Src A"=w461, "Image Dst"=w461, "Image Src B"=w460) -> ("Image Dst Out"=w457:T1)  [unwired: 4 in, 1 out]
                          n202 = call "IMAQ Divide"("Image Src A"=w457, "Constant"=w458, "Image Dst"=w457) -> ()  [unwired: 4 in, 2 out]
                        }
                      }
                    }
                    frame Enabled {
                    }
                  }
                  n203 = local read "开始/暂停"() -> (w440:bool)
                }
                frame "wait heart" {
                  n204 = flat-sequence {
                    frame #0 {
                      n205 = Format Date/Time String() -> (date/time string=w472:string)  [unwired: 3 in]
                      n206 = local read "log"() -> (w467:string)
                      n207 = Concatenate Strings(w472, "\t", "wait heart" ("字符串"), "\r", w467) -> (w469:string)
                      n208 = String Subset(string=w469, length (rest)=1000 ("y")) -> (substring=w468:string)  [unwired: 1 in]
                      n209 = local write "log"(w468) -> ()
                    }
                  }
                  n210 = local read "开始/暂停"() -> (w464:bool)
                }
                frame "wait calibrate" {
                  n211 = local read "开始/暂停"() -> (w474:bool)
                }
                frame "openLightShutter" {
                  n212 = flat-sequence {
                    frame #0 {
                      n213 = local read "address"() -> (w485:i16)
                      n214 = call "Write_para_port2_singalChange.vi"("索引"=1, "布尔"=TRUE, "address"=w485) -> ()  [unwired: 8 in, 1 out]
                    }
                  }
                  n215 = flat-sequence {
                    frame #0 {
                      n216 = Format Date/Time String() -> (date/time string=w484:string)  [unwired: 3 in]
                      n217 = local read "log"() -> (w479:string)
                      n218 = Concatenate Strings(w484, "\t", "open light shutter" ("字符串"), "\r", w479) -> (w481:string)
                      n219 = String Subset(string=w481, length (rest)=1000 ("y")) -> (substring=w480:string)  [unwired: 1 in]
                      n220 = local write "log"(w480) -> ()
                    }
                  }
                  n221 = local read "开始/暂停"() -> (w476:bool)
                }
                frame "closeLightShutter" {
                  n222 = flat-sequence {
                    frame #0 {
                      n223 = local read "address"() -> (w498:i16)
                      n224 = call "Write_para_port2_singalChange.vi"("索引"=1, "布尔"=FALSE, "address"=w498) -> ()  [unwired: 8 in, 1 out]
                    }
                  }
                  n225 = flat-sequence {
                    frame #0 {
                      n226 = Format Date/Time String() -> (date/time string=w497:string)  [unwired: 3 in]
                      n227 = local read "log"() -> (w492:string)
                      n228 = Concatenate Strings(w497, "\t", "close light shutter" ("字符串"), "\r", w492) -> (w494:string)
                      n229 = String Subset(string=w494, length (rest)=1000 ("y")) -> (substring=w493:string)  [unwired: 1 in]
                      n230 = local write "log"(w493) -> ()
                    }
                  }
                  n231 = local read "开始/暂停"() -> (w489:bool)
                }
                frame "writing data" {
                  n232 = while {
                    stop <- w511 continue-if-true
                    n233 = local read "writeing data"() -> (w511:bool)
                    n234 = Wait (ms)(milliseconds to wait=u32 1 ("等待时间（毫秒）")) -> ()  [unwired: 1 out]
                  }
                  n235 = flat-sequence {
                    frame #0 {
                      n236 = Format Date/Time String() -> (date/time string=w510:string)  [unwired: 3 in]
                      n237 = local read "log"() -> (w505:string)
                      n238 = Concatenate Strings(w510, "\t", "writing data" ("字符串"), "\r", w505) -> (w507:string)
                      n239 = String Subset(string=w507, length (rest)=1000 ("y")) -> (substring=w506:string)  [unwired: 1 in]
                      n240 = local write "log"(w506) -> ()
                    }
                  }
                  n241 = local read "开始/暂停"() -> (w502:bool)
                }
              }
            }
            "Stim_ID" <- w317
          }
          n242 = Flush File(refnum=w249) -> (refnum out=w248:refnum<file>)  [unwired: 1 in, 1 out]
          n243 = flat-sequence {
            tunnel: "Pra_DR/R parameter" -> [w280]
            tunnel: w248 -> [w279]
            tunnel: w250 -> [w278]
            frame #0 {
              n244 = local read "Pra_stim ID"() -> (w277:u8[])
              n245 = call "dR_R_ForFile.vi"("DR/R parameter"=w280, "clip ratio"="Pra_clip ratio", "stim ID"=w277, "OnlineMap"="Pra_OnlineMap", "blkIndex"=w278, "BlkFile"=w279) -> ("onLineMapOutput"=w275:T1[])  [unwired: 5 in]
              "onLineMapOutput" <- w275
              n246 = Format Date/Time String() -> (date/time string=w274:string)  [unwired: 3 in]
              n247 = local read "log"() -> (w269:string)
              n248 = call "IMAQ Browser Setup"("Image Ratio"=sgl 1.0, "Browser Info"=T13 {"Browser Size"={"X"=1200, "Y"=256}, "Images per Line"=6, "Background Color"=10066329, "Frame Size"=3, "Frame Style"=enum."Raised"}, "Image In"="browse" ("Image Name")) -> ("Image Browser Out"=w260:T1)  [unwired: 1 in, 3 out]
              n249 = local read "FrameHeight"() -> (w265:i64)
              n250 = local read "FrameWidth"() -> (w266:i64)
              n251 = Concatenate Strings(w274, "\t", "On Line Map" ("字符串"), "\r", w269) -> (w271:string)
              n252 = call "IMAQ Browser Focus Setup"("Focus Color"=u32 16711680, "Image Browser In"=w260) -> ("error out"=w256:errorcluster, "Image Browser Out"=w259:T1)  [unwired: 2 in]
              n253 = String Subset(string=w271, length (rest)=1000 ("y")) -> (substring=w270:string)  [unwired: 1 in]
              n254 = for {
                N: 16 -> [_]
                tunnel: w275 -> [w287] mode=indexing
                tunnel: w266 -> [_]
                tunnel: w265 -> [_]
                tunnel: w259 -> [w292]
                tunnel: w256 -> [_]
                i -> [w293]
                w284 = 3 items=["White", "Black", "Inverted", "Black on White", "White on Black"] ("Color")
                (unwired) u32 13816530 ("BG Color (Transparent)")
                w289 = T4 4 items=["Grayscale (U8)", "Grayscale (I16)", "Grayscale (SGL)", "Complex (CSG)", "RGB (U32)", "HSL (U32)", "RGB (U64)", "Grayscale (U16)"] ("Image Type")
                w295 = "write file data" ("替换字符串(\"\")")
                w298 = T4 0 items=["Grayscale (U8)", "Grayscale (I16)", "Grayscale (SGL)", "Complex (CSG)", "RGB (U32)", "HSL (U32)", "RGB (U64)", "Grayscale (U16)"] ("Image Type")
                n255 = call "IMAQ GetImageInfo"("Image"=w287) -> ("Image Name"=w283:string)  [unwired: 3 in, 7 out]
                n256 = call "IMAQ Cast Image"("Image Type"=w289, "Image Dst"="browseTemp" ("Image Name"), "Image Src"=w287) -> ("Image Dst Out"=w286:T1)  [unwired: 7 in, 1 out]
                n257 = call "IMAQ GetImageInfo"("Image"=w295) -> ("error out"=w296:errorcluster)  [unwired: 3 in, 7 out]
                n258 = case shown="错误" w296 {
                  tunnel: w295 -> [w310 w312]
                  tunnel: [w310 w311] -> w294
                  frame No Error {
                  }
                  frame Error {
                    w313 = T4 0 items=["Grayscale (U8)", "Grayscale (I16)", "Grayscale (SGL)", "Complex (CSG)", "RGB (U32)", "HSL (U32)", "RGB (U64)", "Grayscale (U16)"] ("Image Type")
                    n259 = call "IMAQ Create"("Image Name"=w312, "Image Type"=w313) -> ("New Image"=w311:T1)  [unwired: 3 in, 1 out]
                  }
                }
                n260 = call "IMAQ Draw Text"("String"=w283, "Color"=w284, "Font, Size & Style"=T14 {"Desired Font (Application)"=enum."User-specified Font", "[User-specified Font]"={"Font Name"="arial", "Size"=50, "Strikeout?"=FALSE, "Italic?"=FALSE, "Underline?"=FALSE, "Outline?"=FALSE, "Shadow?"=FALSE, "Bold?"=TRUE, "Rotation Angle"=0.0}, "Horizontal Alignment"=0, "Vertical Alignment"=1}, "Image Dst"=w286, "Image Src"=w286) -> ("Image Dst Out"=w282:T1)  [unwired: 3 in, 3 out]
                n261 = Number To Decimal String(number=w293, width (-)=i16 2 ("宽度(-)")) -> (decimal integer string=w307:string)
                n262 = call <vilib>:"Space Constant.vi"() -> ("String"=w306:string)
                n263 = local read "Pra_文件名"() -> (w309:string)
                n264 = Search and Replace String(replace all?=TRUE ("替换全部？(F)"), input string=w307, search string=w306, replace string="0" ("替换字符串(\"\")")) -> (result string=w302:string)  [unwired: 4 in, 3 out]
                n265 = call "IMAQ Browser Insert"("Image Browser In"=w292, "Image to Add"=w282) -> ("Image Browser Out"=w291:T1)  [unwired: 5 in, 4 out]
                n266 = call "IMAQ WindDraw"("Window Number (0...15)"=0, "Image"=w291) -> ()  [unwired: 8 in, 2 out]
                n267 = local read "Pra_Blk目录"() -> (w297:path)
                n268 = Concatenate Strings(w309, "_" ("字符串"), w302, ".bmp" ("字符串")) -> (w300:string)
                n269 = call "IMAQ Cast Image"("Image Type"=w298, "Image Dst"=w294, "Image Src"=w287) -> ("Image Dst Out"=w290:T1)  [unwired: 7 in, 1 out]
                n270 = Build Path(base path=w297, name or relative path=w300) -> (appended path=w299:path)
                n271 = call-poly "IMAQ Write File 2"("File Path"=w299, "Image"=w290) -> ()  [unwired: 8 in, 2 out]
              }
              n272 = local write "log"(w270) -> ()
            }
          }
        }
        frame Error {
          n273 = local write "开始/暂停"(TRUE ("开始/暂停")) -> ()
          n274 = One Button Dialog(message="blk exist, please change the file name" ("消息")) -> ()  [unwired: 1 in, 1 out]
        }
      }
      "block" <- w234
    }
    n275 = Array Size(array="Pra_stim ID") -> (size(s)=w204:i32)
    n276 = local write "Stimuli"(w204) -> ()
    n277 = property on="Pra_bin" class="Enum (严格)"("DisabledEnum"=w201) -> ()  [unwired: 2 in, 2 out]
    n278 = property on="SaveParameter" class="Bool"("DisabledEnum"=w201) -> ()  [unwired: 2 in, 2 out]
    n279 = property on="Pra_binType" class="Enum (严格)"("DisabledEnum"=w201) -> ()  [unwired: 2 in, 2 out]
    n280 = local read "停止循环"() -> (w210:bool)
  }
  n281 = local write "FrameWidth"(w19) -> ()
  n282 = local write "FrameHeight"(w18) -> ()
  n283 = node-c288() -> (w64:T15)
  n284 = timed-loop {
    tunnel: [w531] -> w59
    tunnel: [w553] -> w8
    tunnel: w16 -> [w532]
    tunnel: w4 -> [w552]
    tunnel: w5 -> [w551]
    tunnel: [w550] -> w44
    timing: w64 -> [_]
    timing-out: [_] -> w63
    tunnel: w40 -> [w541]
    tunnel: w12 -> [w536]
    tunnel: w35 -> [w546]
    tunnel: w31 -> [_]
    tunnel: w32 -> [w545]
    tunnel: w29 -> [w544]
    shift-right: [w539] -> _
    shift-left: 1 -> [w540]
    shift-right: [w538] -> _
    shift-left: w24 -> [w537]
    tunnel: w21 -> [w534]
    tunnel: w20 -> [w533]
    tunnel: w19 -> [w529]
    tunnel: w18 -> [w528]
    tunnel: "Pra_binType" -> [w527]
    shift-right: [w521] -> _
    shift-left: _ -> [w525]
    shift-right: [w522] -> _
    shift-left: _ -> [w520]
    tunnel: w13 -> [w519]
    shift-right: [w518] -> _
    shift-left: _ -> [w517]
    tunnel: [w516] -> w1
    i -> [w523]
    stop <- w547 stop-if-true
    n285 = node-c288() -> (→"循环持续时间":i64)  [unwired: 1 in]
    n286 = flat-sequence {
      frame #0 {
      }
      frame #1 {
        n287 = event shown="[3] \"LoadParameter\": 值改变" {
          selector: _ -> [_ _ _ _]
          dyn-events: _ -> [_ _ _ _]
          timeout: 0 -> [_ _ _ _]
          event Timeout {
            n288 = event-data() -> ()  [unwired: 1 in, 2 out]
          }
          event "停止": Value Change {
            n289 = event-data() -> ("NewVal"=w629:bool)  [unwired: 1 in, 1 out]
            n290 = case shown="真" w629 {
              selector: w629 -> [_ w631]
              tunnel: [FALSE w631] -> _
              frame False {
              }
              frame True {
                n291 = local write "开始/暂停"(w631) -> ()
                "停止循环" <- w631
              }
            }
          }
          event "SaveParameter": Value Change {
            n292 = event-data() -> ()  [unwired: 1 in, 1 out]
            n293 = call "文件对话框"("prompt"="SaveParameterTo", "pattern (all files)"="*.prmf", "pattern label"="Flowbit") -> ("selected path"=w633:path, "error out"=w635:errorcluster)  [unwired: 9 in, 2 out]
            n294 = case shown="无错误" w635 {
              tunnel: w633 -> [w638 _]
              frame No Error {
                n295 = control-ref of="本VI"() -> (w642:refnum<vi>)
                n296 = invoke class="VI" method="Ctrl Val.Get All"(reference=w642, "Controls"=TRUE ("输入控件")) -> ("Get All Control Values Variant"=w641:cluster{"Name":string, "Variant Data":variant}[])  [unwired: 2 in, 3 out]
                n297 = for {
                  tunnel: w641 -> [w646] mode=indexing
                  shift-right: [w645] -> w639
                  shift-left: cluster{"Name":string, "Variant Data":variant}[] [] -> [w644]
                  i -> [w643]
                  n298 = Unbundle By Name(w646) -> ("Name"=w651:string)
                  n299 = String Subset(string=w651, length (rest)=4 ("长度（剩余）")) -> (substring=w649:string)  [unwired: 1 in]
                  n300 = Equal?(x=w649, y="Pra_") -> (x = y?=w647:bool)
                  n301 = case shown="真" w647 {
                    tunnel: w646 -> [_ w656]
                    tunnel: [w652 w655] -> w645
                    tunnel: w644 -> [w652 w654]
                    tunnel: w643 -> [_ w653]
                    frame False {
                    }
                    frame True {
                      n302 = case shown="0" w653 {
                        tunnel: w656 -> [w658 w661]
                        tunnel: [w657 w660] -> w655
                        tunnel: w654 -> [_ w659]
                        frame 0 {
                          n303 = Build Array(w658) -> (w657:cluster{"Name":string, "Variant Data":variant}[])
                        }
                        frame 1, Default {
                          n304 = Build Array (concatenate)(w659, w661) -> (w660:cluster{"Name":string, "Variant Data":variant}[])
                        }
                      }
                    }
                  }
                }
                n305 = Write to Binary File(file (use dialog)=w638, data=w639) -> ()  [unwired: 4 in, 3 out]
              }
              frame Error {
              }
            }
          }
          event "LoadParameter": Value Change {
            n306 = event-data() -> ()  [unwired: 1 in, 1 out]
            n307 = call "文件对话框2"("prompt"="LoadParameter", "pattern (all files)"="*.prmf", "pattern label"="Flowbit") -> ("selected path"=w662:path, "error out"=w663:errorcluster)  [unwired: 9 in, 2 out]
            n308 = case shown="无错误" w663 {
              tunnel: w662 -> [w671 _]
              tunnel: [w667 _] -> _
              frame No Error {
                n309 = Read from Binary File(5:cluster{"Name":string, "Variant Data":variant}[] [], 11:w671) -> (2:w668:cluster{"Name":string, "Variant Data":variant}[])  [unwired: 4 in, 3 out]
                n310 = control-ref of="本VI"() -> (w669:refnum<vi>)
                n311 = for {
                  tunnel: w669 -> [w677]
                  tunnel: w668 -> [w676] mode=indexing
                  tunnel: [w672] -> w667 mode=indexing
                  n312 = Unbundle By Name(w676) -> ("Name"=w675:string, "Variant Data"=w674:variant)
                  n313 = invoke class="VI" method="Ctrl Val.Set"(reference=w677, "Control Name"=w675, "Value"=w674) -> (error out=w673:errorcluster)  [unwired: 2 in, 4 out]
                  n314 = call <vilib>:"Clear Errors.vi"("error in (no error)"=w673) -> ("error out"=w672:errorcluster)  [unwired: 6 in]
                }
              }
              frame Error {
              }
            }
          }
        }
      }
    }
    n315 = Get Queue Status(queue=w536) -> (queue out=w535:refnum<queue>, # elements in queue=→"队列中元素数量":i32)  [unwired: 2 in, 6 out]
    n316 = case shown="\"2*2\"" "Pra_bin" {
      tunnel: w534 -> [_ w615]
      tunnel: w533 -> [_ w610]
      tunnel: w532 -> [w608 w614]
      tunnel: [w608 w613] -> w531
      tunnel: w529 -> [_ w619]
      tunnel: w528 -> [_ w616]
      tunnel: w527 -> [_ w609]
      frame "1*1", Default {
      }
      frame "2*2" {
        n317 = Divide(x=w619, y=2) -> (x/y=w612:dbl)
        n318 = Divide(x=w616, y=2) -> (x/y=w611:dbl)
        n319 = local write "FrameWidth"(w612) -> ()
        n320 = case shown="\"Resample\"" w609 {
          tunnel: w615 -> [_ w626]
          tunnel: w614 -> [w621 w627]
          tunnel: [w620 w623] -> w613
          tunnel: w612 -> [_ w625]
          tunnel: w611 -> [_ w624]
          tunnel: w610 -> [_ w622]
          frame "Extract", Default {
            n321 = call "Bin2.vi"("Image Src"=w621) -> ("Image"=w620:T1)  [unwired: 10 in]
          }
          frame "Resample" {
            n322 = call "IMAQ Resample"("X Resolution"=w625, "Y Resolution"=w624, "Interpolation Type"=w622, "Image Dst"=w626, "Image Src"=w627) -> ("Image Dst Out"=w623:T1)  [unwired: 5 in, 1 out]
          }
        }
        n323 = local write "FrameHeight"(w611) -> ()
      }
    }
    n324 = local read "Recording"() -> (w521:bool)
    n325 = case shown="真" w521 {
      tunnel: w535 -> [w554 w566]
      tunnel: w531 -> [_ w571]
      tunnel: w541 -> [_ w570]
      tunnel: w540 -> [_ w562]
      tunnel: [1 w567] -> w539
      tunnel: w537 -> [_ w563]
      tunnel: [u32[][] [] w565] -> w538
      tunnel: [w555 w559] -> w518
      tunnel: w517 -> [_ w560]
      tunnel: [w554 w558] -> w516
      frame False {
        n326 = local read "Pra_FramesPerStim"() -> (w555:i64)
      }
      frame True {
        n327 = call "IMAQ Copy"("Image Dst"=w570, "Image Src"=w571) -> ("Image Dst Out"=w569:T1)  [unwired: 4 in, 1 out]
        n328 = call "IMAQ ImageToArray"("Image"=w569) -> ("Image Pixels (I16)"=w564:i16[][])  [unwired: 3 in, 4 out]
        n329 = Greater?(x="Pra_FrameBin", y=w562) -> (0:w568:bool)
        n330 = case shown="假" w568 {
          tunnel: w562 -> [_ w592]
          tunnel: [1 w591] -> w567
          tunnel: w566 -> [w581 w589]
          tunnel: [u32[][] [] w594] -> w565
          tunnel: w564 -> [w580 w596]
          tunnel: w563 -> [w579 w595]
          tunnel: w562 -> [_ w593]
          tunnel: "Pra_FrameBin" -> [w576 _]
          tunnel: w560 -> [w575 w590]
          tunnel: [w573 w590] -> w559
          tunnel: [w572 w589] -> w558
          frame False {
            n331 = case shown="0, 默认" w576 {
              tunnel: w580 -> [w586 w588]
              tunnel: w579 -> [w585 _]
              tunnel: [w584 w587] -> w577
              frame 0, Default {
                n332 = Add(x=w586, y=w585) -> (x+y=w584:u32[][])
              }
              frame 1 {
                n333 = To Unsigned Long Integer(number=w588) -> (unsigned 32bit integer=w587:u32[][])
              }
            }
            n334 = Decrement(x=w575) -> (x-1=w573:i64)
            n335 = Less Or Equal To 0?(x=w573) -> (x <= 0?=w574:bool)
            n336 = case shown="真" w574 {
              frame False {
              }
              frame True {
                n337 = local write "Recording"(FALSE ("Recording")) -> ()
              }
            }
            n338 = Enqueue Element(queue=w581, element=w577) -> (queue out=w572:refnum<queue>)  [unwired: 2 in, 2 out]
          }
          frame True {
            n339 = case shown="1" w593 {
              tunnel: w596 -> [w597 w600]
              tunnel: w595 -> [_ w599]
              tunnel: [w597 w598] -> w594
              frame 1 {
              }
              frame 0, Default {
                n340 = Add(x=w600, y=w599) -> (x+y=w598:u32[][])
              }
            }
            n341 = Increment(x=w592) -> (x+1=w591:i32)
          }
        }
      }
    }
    n342 = Not Equal?(x=w521, y=w525) -> (x != y?=w524:bool)
    n343 = case shown="假" "热图" {
      tunnel: w546 -> [w684 w692]
      tunnel: w531 -> [w678 w690]
      tunnel: [w678 w689] -> w543
      tunnel: w545 -> [_ w687]
      tunnel: w544 -> [_ w686]
      tunnel: w519 -> [w682 _]
      frame False {
        w683 = T4 0 items=["Grayscale (U8)", "Grayscale (I16)", "Grayscale (SGL)", "Complex (CSG)", "RGB (U32)", "HSL (U32)", "RGB (U64)", "Grayscale (U16)"] ("Image Type")
        n344 = call "IMAQ Copy"("Image Dst"=w684, "Image Src"=w678) -> ("Image Dst Out"=w681:T1)  [unwired: 4 in, 1 out]
        n345 = call "IMAQ Divide"("Image Src A"=w681, "Constant"=sgl 16.0, "Image Dst"=w681) -> ("Image Dst Out"=w679:T1)  [unwired: 4 in, 1 out]
        n346 = call "IMAQ Cast Image"("Image Type"=w683, "Image Dst"=w682, "Image Src"=w679) -> ()  [unwired: 7 in, 2 out]
      }
      frame True {
        w688 = T4 4 items=["Grayscale (U8)", "Grayscale (I16)", "Grayscale (SGL)", "Complex (CSG)", "RGB (U32)", "HSL (U32)", "RGB (U64)", "Grayscale (U16)"] ("Image Type")
        n347 = call "IMAQ Copy"("Image Dst"=w692, "Image Src"=w690) -> ("Image Dst Out"=w691:T1)  [unwired: 4 in, 1 out]
        n348 = call "IMAQ Divide"("Image Src A"=w691, "Constant"=sgl 256.0, "Image Dst"=w691) -> ("Image Dst Out"=w685:T1)  [unwired: 4 in, 1 out]
        n349 = call "IMAQ Cast Image"("Image Type"=w688, "Lookup Table"=w686, "Image Dst"=w687, "Image Src"=w685) -> ("Image Dst Out"=w689:T1)  [unwired: 6 in, 1 out]
      }
    }
    "Image 2" <- w543
    n350 = case shown="真" w524 {
      tunnel: w523 -> [_ w602]
      tunnel: [w601 w602] -> w522
      tunnel: w520 -> [w601 w603]
      tunnel: w521 -> [_ w604]
      tunnel: w520 -> [_ _]
      frame False {
      }
      frame True {
        n351 = case shown="假" w604 {
          tunnel: w603 -> [w606 _]
          tunnel: w602 -> [w605 _]
          frame False {
            n352 = Subtract(x=w605, y=w606) -> (x-y=→"grabLoop":i32)
          }
          frame True {
          }
        }
      }
    }
    n353 = local read "停止循环"() -> (w547:bool)
    n354 = call <vilib>:"Wait For Frame.vi"("error in (no error)"=w552, "Timeout (mS)"=u32 5000, "RefBrdIn"=w551) -> ("error out"=w553:errorcluster, "RefBrdOut"=w550:u32)  [unwired: 7 in]
    n355 = node-c288() -> ()  [unwired: 1 in, 1 out]
  }
  n356 = node-c288(w63) -> ()  [unwired: 1 out]
  n357 = call "IMAQ WindClose"("Close All Windows (False)"=TRUE, "error in (no error)"=w8) -> ("error out"=w7:errorcluster)  [unwired: 4 in]
  n358 = call <vilib>:"Stop.vi"("error in (no error)"=w7, "Image In"=w59, "RefBrdIn"=w44) -> ("error out"=w55:errorcluster, "Image"=w58:T1, "RefBrdOut"=w43:u32)  [unwired: 6 in]
  n359 = call <vilib>:"Cleanup.vi"("error in (no error)"=w55, "Image In"=w58, "RefBrdIn"=w43) -> ("error out"=w56:errorcluster, "Image"=w57:T1, "RefBrdOut"=w42:u32)  [unwired: 6 in]
  n360 = call <vilib>:"Close.vi"("error in (no error)"=w56, "RefBrdIn"=w42) -> ("error out"=w41:errorcluster)  [unwired: 8 in, 1 out]
  n361 = call "Imaq Dispose"("Image"=w57, "error in (no error)"=w41) -> ("error out"=w3:errorcluster)  [unwired: 4 in]
  n362 = flat-sequence {
    tunnel: w3 -> [w699]
    tunnel: [w698] -> w2
    tunnel: w1 -> [w697]
    tunnel: w2 -> [_]
    frame #0 {
      n363 = Flush Queue(queue=w697, error in (no error)=w699) -> (error out=w698:errorcluster)  [unwired: 2 out]
    }
    frame #1 {
      (unwired) 0.0 ("Output Voltage (V) (0.0)")
    }
    frame #2 {
      n364 = Stop(stop? (T)=TRUE ("停止？(T)")) -> ()
    }
  }
